vi "SA_RBW.vi"(0 "Session In":refnum<visa-resource-name>="GPIB0::16::INSTR", 7 "RBW(Hz)":string="30", 11 "error in":errorcluster {"code" format="%.0x"}, 12 "RO (T)":bool, 13 "RBW AUTO":i32(ring) items=["RBW AUTO OFF", "RBW AUTO ON"]) -> (4 "Session Out":refnum<visa-resource-name>, 8 "RBW Read":dbl, 10 "AUTO (read)":string, 14 "RBW coerced (T)":bool, 15 "error out":errorcluster {"code" format="%.0x"})   [LabVIEW 2018]
doc: "Launches the Instrument I/O Assistant, which you can use to communicate with message-based instruments and graphically parse the response. For example you can communicate with an instrument that uses a serial, Ethernet, or GPIB interface."
panel:
  in  "Timeout":u32=3000
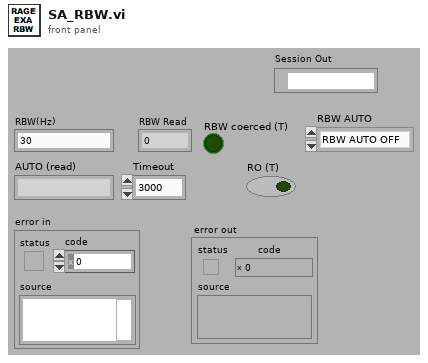
[diagram p1: front panel]
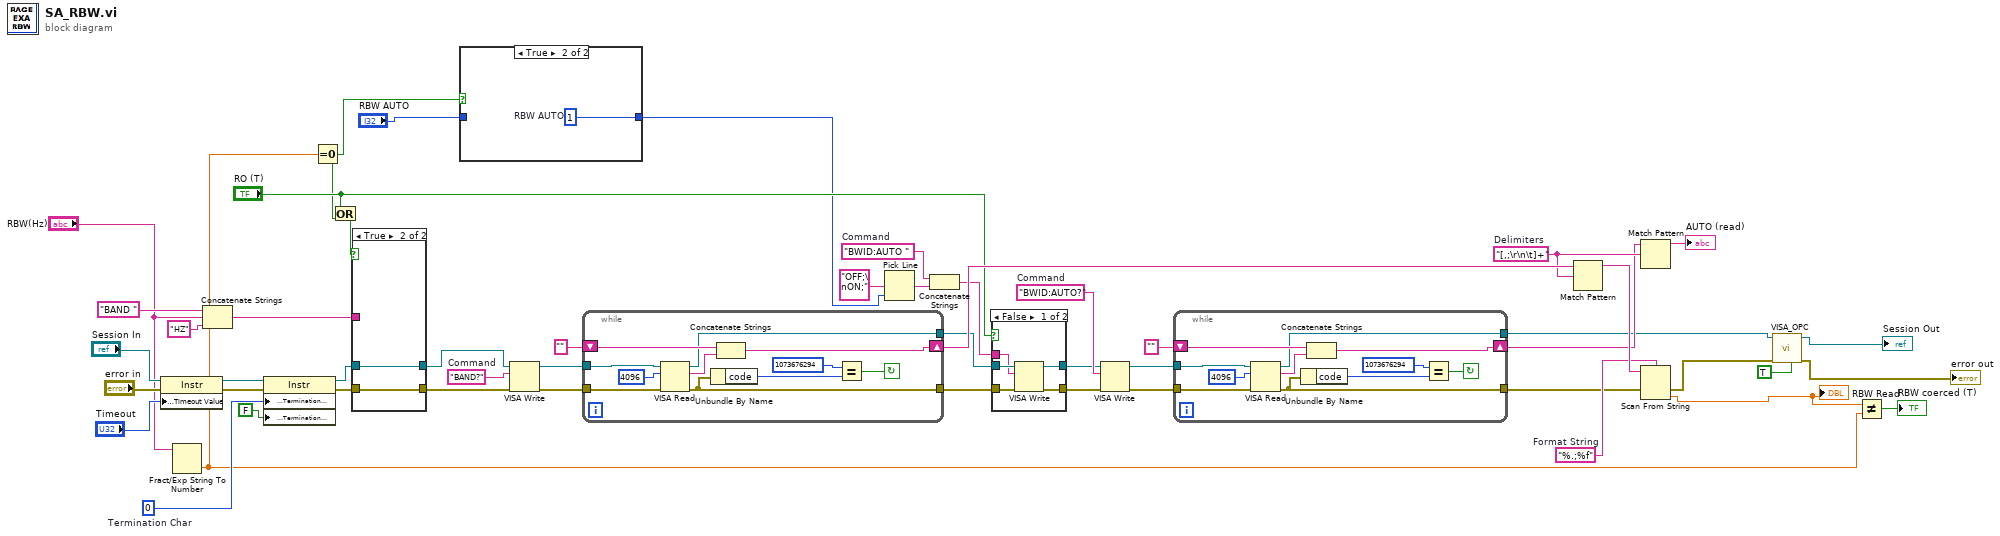
[diagram p0: block diagram]
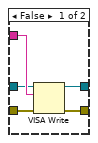
[diagram p4: hidden frame]
diagram:
  w15 = "BWID:AUTO "  # Command
  w28 = "BWID:AUTO?"  # Command
  w20 = "[,;\r\n\t]+"  # Delimiters
  w34 = "%.;%f"  # Format String
  w37 = "BAND?"  # Command
  w46 = u8 0  # Termination Char
  n1 = property class="Instr"(reference="Session In", error in="error in", "General Settings:Timeout Value"="Timeout") -> (reference out=w45:refnum<visa-resource-name>, error out=w48:errorcluster)
  n2 = Fract/Exp String To Number(string="RBW(Hz)") -> (number=w10:dbl)  [unwired: 3 in, 1 out]
  n3 = Concatenate Strings("BAND " ("staticText"), "RBW(Hz)", "HZ" ("string")) -> (w41:string)
  n4 = property class="Instr"(reference=w45, error in=w48, "Message Based Settings:Termination Character"=w46, "Message Based Settings:Termination Character Enable"=FALSE ("enable")) -> (reference out=w24:refnum<visa-resource-name>, error out=w47:errorcluster)
  n5 = Equal To 0?(x=w10) -> (x = 0?=w7:bool)
  n6 = Or(x="RO (T)", y=w7) -> (x .or. y?=w9:bool)
  n7 = case shown="True" w9 {
    tunnel: w47 -> [w56 w57]
    tunnel: [w55 w57] -> w42
    tunnel: w41 -> [w54 _]
    tunnel: w24 -> [w53 w58]
    tunnel: [w52 w58] -> w33
    frame False {
      n8 = VISA Write(VISA resource name=w53, write buffer=w54, error in (no error)=w56) -> (VISA resource name out=w52:refnum<visa-resource-name>, error out=w55:errorcluster)  [unwired: 1 out]
    }
    frame True {
    }
  }
  n9 = case shown="True" w7 {
    tunnel: [w59 w60] -> w16
    tunnel: "RBW AUTO" -> [w59 _]
    frame False {
    }
    frame True {
      w60 = 1  # RBW AUTO
    }
  }
  n10 = VISA Write(VISA resource name=w33, write buffer=w37, error in (no error)=w42) -> (VISA resource name out=w40:refnum<visa-resource-name>, error out=w39:errorcluster)  [unwired: 1 out]
  n11 = while {
    tunnel: w40 -> [w68]
    shift-right: [w63] -> w36
    shift-left: "" -> [w67]
    tunnel: w39 -> [w65]
    tunnel: [w62] -> w22
    tunnel: [w61] -> w21
    stop <- w64 continue-if-true
    n12 = VISA Read(VISA resource name=w68, byte count=u32 4096 ("byte count (0)"), error in (no error)=w65) -> (VISA resource name out=w62:refnum<visa-resource-name>, read buffer=w66:string, error out=w61:errorcluster)  [unwired: 1 out]
    n13 = Unbundle By Name(w61) -> ("code"=w70:i32)
    n14 = Concatenate Strings(w67, w66) -> (w63:string)
    n15 = Equal?(x=1073676294, y=w70) -> (x = y?=w64:bool)
  }
  n16 = Pick Line(multi-line string="OFF;\nON;" ("write buffer"), line index=w16) -> (output string=w14:string)  [unwired: 1 in]
  n17 = Concatenate Strings(w15, w14) -> (w13:string)
  n18 = case shown="False" "RO (T)" {
    tunnel: w21 -> [w73 w77]
    tunnel: [w76 w77] -> w26
    tunnel: w22 -> [w75 w78]
    tunnel: [w74 w78] -> w25
    tunnel: w13 -> [w72 _]
    frame False {
      n19 = VISA Write(VISA resource name=w75, write buffer=w72, error in (no error)=w73) -> (VISA resource name out=w74:refnum<visa-resource-name>, error out=w76:errorcluster)  [unwired: 1 out]
    }
    frame True {
    }
  }
  n20 = VISA Write(VISA resource name=w25, write buffer=w28, error in (no error)=w26) -> (VISA resource name out=w29:refnum<visa-resource-name>, error out=w30:errorcluster)  [unwired: 1 out]
  n21 = while {
    tunnel: w29 -> [w86]
    shift-right: [w80] -> w19
    shift-left: "" -> [w85]
    tunnel: w30 -> [w83]
    tunnel: [w82] -> w12
    tunnel: [w79] -> w4
    stop <- w81 continue-if-true
    n22 = VISA Read(VISA resource name=w86, byte count=u32 4096 ("byte count (0)"), error in (no error)=w83) -> (VISA resource name out=w79:refnum<visa-resource-name>, read buffer=w84:string, error out=w82:errorcluster)  [unwired: 1 out]
    n23 = Unbundle By Name(w82) -> ("code"=w88:i32)
    n24 = Concatenate Strings(w85, w84) -> (w80:string)
    n25 = Equal?(x=1073676294, y=w88) -> (x = y?=w81:bool)
  }
  n26 = Match Pattern(string=w36, regular expression=w20) -> (before substring=w35:string)  [unwired: 1 in, 3 out]
  n27 = Match Pattern(string=w19, regular expression=w20) -> (before substring=→"AUTO (read)":string)  [unwired: 1 in, 3 out]
  n28 = Scan From String(format string=w34, input string=w35, error in=w12) -> (error out=w3:errorcluster, output 1=w6:dbl)  [unwired: 2 in, 2 out]
  "RBW Read" <- w6
  n29 = call "VISA_OPC.vi"("OPC(T)"=TRUE ("OPC?(T)"), "error in"=w3, "Session In"=w4) -> ("error out"=→"error out":errorcluster, "Session Out"=→"Session Out":refnum<visa-resource-name>)  [unwired: 6 in, 1 out]
  n30 = Not Equal?(x=w6, y=w10) -> (x != y?=→"RBW coerced (T)":bool)
